vi "Main.vi"() -> ()   [LabVIEW 2019, in "OCV4.lvlib" / "OCV4.lvclass"]
uses:
  OCV4.lvclass
  typeDefs/Server State Data.ctl
  OCV4.lvclass/OCV4.ctl
panel:
  in  "Enable Async Mode":bool
  out "Numeric":i32
  in  "Stop":bool
  in  "Server Address":string="0.0.0.0:50051"
  in  "Server Certificate File (.crt)":path
  in  "Server Key File (.key)":path
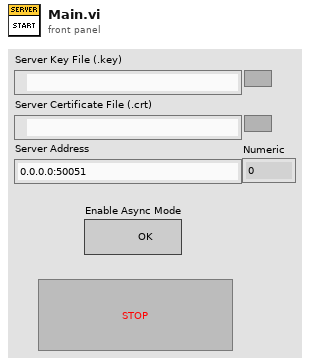
[diagram p1: front panel]
types:
  T1 = typedef "OCV4.lvlib/OCV4.lvclass/Server State Data.ctl" = cluster{"Data":string}
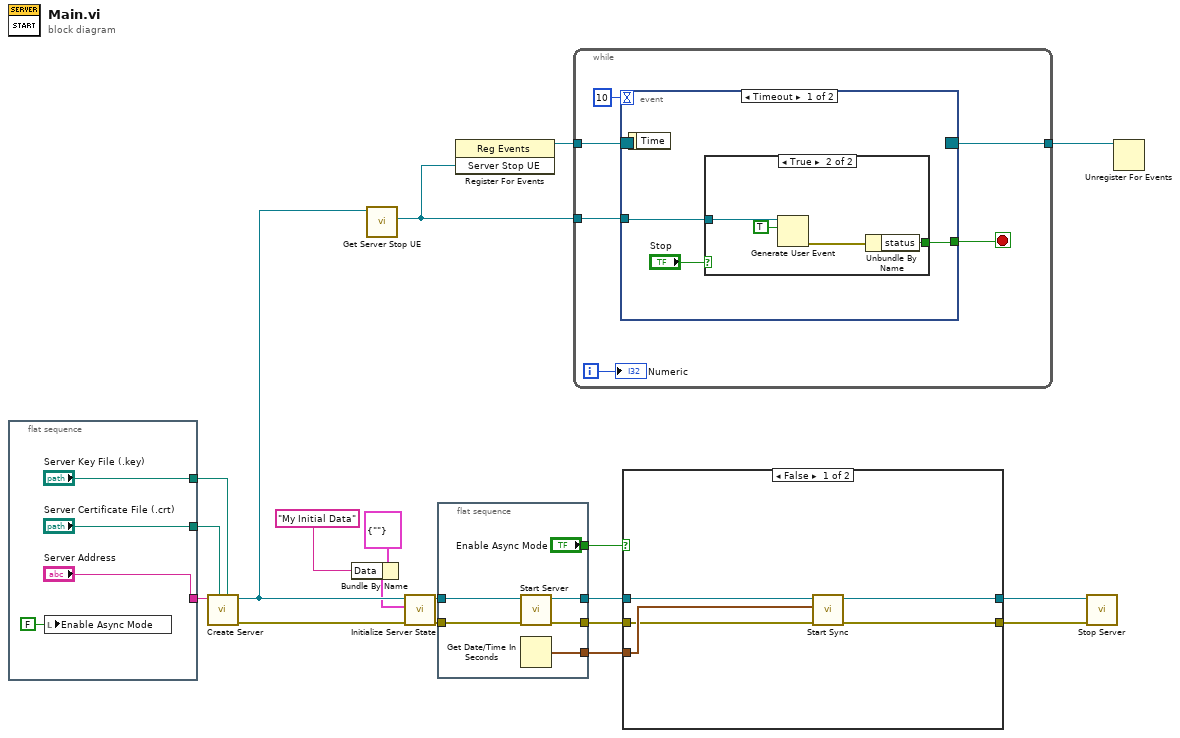
[diagram p0: block diagram]
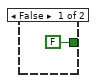
[diagram p2: hidden frame]
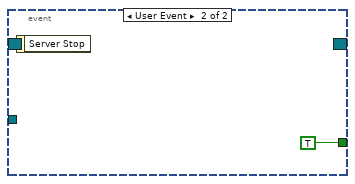
[diagram p3: hidden frame]
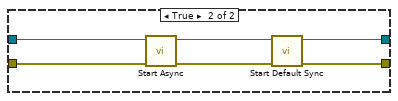
[diagram p4: hidden frame]
diagram:
  n1 = flat-sequence {
    tunnel: ["Server Key File (.key)"] -> w15
    tunnel: ["Server Certificate File (.crt)"] -> w14
    tunnel: ["Server Address"] -> w13
    frame #0 {
      n2 = local write "Enable Async Mode"(FALSE ("Enable Async Mode")) -> ()
    }
  }
  n3 = call "Create Server.vi"("Server Key File (.key)"=w15, "Server Certificate File (.crt)"=w14, "Server Address"=w13) -> ("error out"=w8:errorcluster, "gRPC Server out"=w5:refnum<class "OCV4.lvclass">)  [unwired: 7 in]
  n4 = Bundle By Name(cluster=T1 {"Data"=""} ("Initial State"), "Data"="My Initial Data") -> (w3:T1)
  n5 = call "Get Server Stop UE.vi"("OOP Server in"=w5) -> ("Server Stop UE"=w9:refnum<user-event>)  [unwired: 9 in, 1 out]
  n6 = call "Initialize Server State.vi"("error in (no error)"=w8, "Initial State"=w3, "gRPC Server in"=w5) -> ("error out"=w7:errorcluster, "gRPC Server out"=w6:refnum<class "OCV4.lvclass">)  [unwired: 7 in]
  n7 = flat-sequence {
    tunnel: [w29] -> w19
    tunnel: [w28] -> w18
    tunnel: ["Enable Async Mode"] -> w12
    tunnel: w7 -> [w26]
    tunnel: w6 -> [w25]
    tunnel: [w24] -> w1
    frame #0 {
      n8 = call "Start Server.vi"("error in (no error)"=w26, "gRPC Server in"=w25) -> ("error out"=w29:errorcluster, "gRPC Server out"=w28:refnum<class "OCV4.lvclass">)  [unwired: 8 in]
      n9 = Get Date/Time In Seconds() -> (seconds since 1Jan1904=w24:timestamp)
    }
  }
  n10 = register-events(w9) -> (reference out=w11:refnum<event-registration>)  [unwired: 2 in, 1 out]
  n11 = while {
    tunnel: w9 -> [w35]
    tunnel: w11 -> [w34]
    tunnel: [w32] -> w10
    i -> [w31]
    stop <- w33 stop-if-true
    n12 = event shown="[0] Timeout" {
      selector: w34 -> [_ _]
      dyn-events: [_ _] -> w32
      timeout: 10 -> [_ _]
      tunnel: w35 -> [w38 _]
      tunnel: [w37 TRUE] -> w33
      event Timeout {
        n13 = event-data() -> ()  [unwired: 1 in, 1 out]
        n14 = case shown="True" "Stop" {
          tunnel: w38 -> [_ w41]
          tunnel: [FALSE ("status") w40] -> w37
          frame False {
          }
          frame True {
            n15 = Generate User Event(user event=w41, event data cluster=TRUE ("event data")) -> (error out=w42:errorcluster)  [unwired: 2 in, 1 out]
            n16 = Unbundle By Name(w42) -> ("status"=w40:bool)
          }
        }
      }
      event User Event {
        n17 = event-data() -> ()  [unwired: 1 in, 1 out]
      }
    }
    "Numeric" <- w31
  }
  n18 = case shown="False" w12 {
    tunnel: w19 -> [w45 w55]
    tunnel: w18 -> [w46 w54]
    tunnel: [w49 w51] -> w17
    tunnel: [w48 w50] -> w16
    tunnel: w1 -> [w47 _]
    frame False {
      n19 = call "Start Sync.vi"("error in (no error)"=w45, "current time"=w47, "gRPC Server in"=w46) -> ("error out"=w49:errorcluster, "gRPC Server out"=w48:refnum<class "OCV4.lvclass">)  [unwired: 7 in]
    }
    frame True {
      n20 = call "Start Async.vi"("error in (no error)"=w55, "gRPC Server in"=w54) -> ("error out"=w52:errorcluster, "gRPC Server out"=w53:refnum<class "OCV4.lvclass">)  [unwired: 8 in]
      n21 = call "Start Default Sync.vi"("error in (no error)"=w52, "gRPC Server in"=w53) -> ("error out"=w51:errorcluster, "gRPC Server out"=w50:refnum<class "OCV4.lvclass">)  [unwired: 8 in]
    }
  }
  n22 = call "Stop Server.vi"("error in (no error)"=w17, "gRPC Server in"=w16) -> ()  [unwired: 9 in, 1 out]
  n23 = Unregister For Events(event registration refnum=w10) -> ()  [unwired: 1 in, 1 out]
